vi "Joystick Toggle.vi"(4 "Max":dbl, 6 "Min":dbl, 9 "Value":dbl, 11 "Range":dbl) -> (1 "Output":dbl)   [LabVIEW 2018]
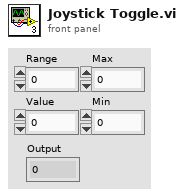
[diagram p1: front panel]
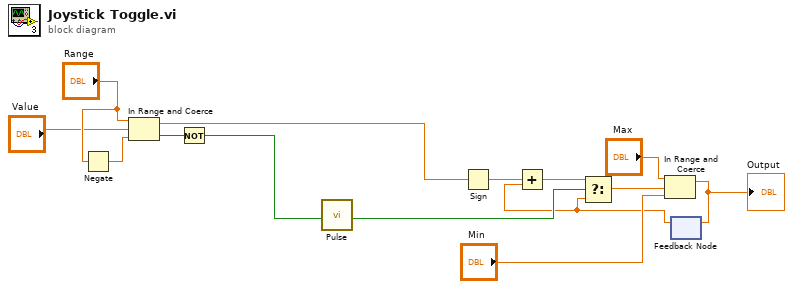
[diagram p0: block diagram]
diagram:
  n1 = Negate(x="Range") -> (-x=w12:dbl)
  n2 = In Range and Coerce(upper limit="Range", x="Value", lower limit=w12) -> (coerced(x)=w6:dbl, In Range?=w13:bool)
  n3 = Not(x=w13) -> (.not. x?=w14:bool)
  n4 = call "Pulse.vi"("Input"=w14) -> ("Output"=w8:bool)  [unwired: 10 in]
  n5 = Sign(1:w6) -> (0:w9:dbl)
  n6 = feedback #1() -> (w1:dbl)  [unwired: 1 in]
  n7 = Add(x=w9, y=w1) -> (x+y=w7:dbl)
  n8 = Select(t=w7, s=w8, f=w1) -> (s? t:f=w5:dbl)
  n9 = In Range and Coerce(upper limit="Max", x=w5, lower limit="Min") -> (coerced(x)=w2:dbl)  [unwired: 1 out]
  "Output" <- w2
  n10 = feedback-in #1(w2) -> ()
